vi "Error Handler.vi"(7 "function (unspecified)":T1, 8 "error in (no error)":errorcluster, 11 "errno":T2) -> (0 "error out":errorcluster)   [LabVIEW 2013, in "Linux RT IPC.lvlib" / "Pipes.lvlib"]
uses:
  Pipes.lvlib
  <vilib>/NI/NI Linux RT Errno/Controls/Public/errno.ctl
  Controls/functions.ctl
  <vilib>/NI/NI Linux RT Errno/Linux Errno.lvlib
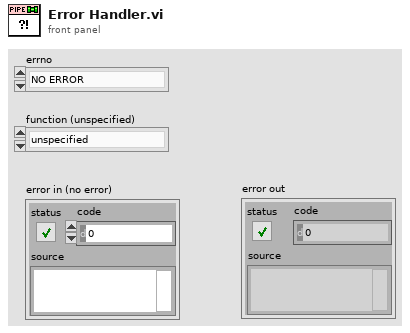
[diagram p1: front panel]
types:
  T1 = typedef "Linux RT IPC.lvlib/Pipes.lvlib/functions.ctl" = enum16{"unspecified", "mkfifo", "open", "read", "write", "close", "unlink"}
  T2 = typedef "Linux Errno.lvlib/errno.ctl" = enum16{"NO ERROR", "EPERM", "ENOENT", "ESRCH", "EINTR", "EIO", "ENXIO", "E2BIG", "ENOEXEC", "EBADF", "ECHILD", "EAGAIN", "ENOMEM", "EACCES", "EFAULT", "ENOTBLK", "EBUSY", "EEXIST", "EXDEV", "ENODEV", "ENOTDIR", "EISDIR", "EINVAL", "ENFILE", "EMFILE", "ENOTTY", "ETXTBSY", "EFBIG", "ENOSPC", "ESPIPE", "EROFS", "EMLINK", "EPIPE", "EDOM", "ERANGE", "EDADLK", "ENAMETOOLONG", "ENOLCK", "ENOSYS", "ENOTEMPTY", "ELOOP", "EWOULDBLOCK", "ENOMSG", "EIDRM", "ECHRNG", "EL2NSYNC", "EL3HLT", "EL3RST", "ELNRNG", "EUNATCH", "ENOCSI", "EL2HLT", "EBADE", "EBADR", "EXFULL", "ENOANO", "EBADRQC", "EBADSLT", "EDEADLOCK", "EBFONT", "ENOSTR", "ENODATA", "ETIME", "ENOSR", "ENONET", "ENOPKG", "EREMOTE", "ENOLINK", "EADV", "ESRMNT", "ECOMM", "EPROTO", "EMULTIHOP", "EDOTDOT", "EBADMSG", "EOVERFLOW", "ENOTUNIQ", "EBADFD", "EREMCHG", "ELIBACC", "ELIBBAD", "ELIBSCN", "ELIBMAX", "ELIBEXEC", "ELISEQ", "ERESTART", "ESTRPIPE", "EUSERS", "ENOTSOCK", "EDESTADDRREQ", "EMSGSIZE", "EPROTOTYPE", "ENOPROTOOPT", "EPROTONOSUPPORT", "ESOCKTNOSUPPORT", "EOPNOTSUPP", "EPFNOSUPPORT", "EAFNOSUPPORT", "EADDRINUSE", "EADDRNOTAVAIL", "ENETDOWN", "ENETUNREACH", "ENETRESET", "ECONNABORTED", "ECONNRESET", "ENOBUFS", "EISCONN", "ENOTCONN", "ESHUTDOWN", "ETOOMANYREFS", "ETIMEDOUT", "ECONNREFUSED", "EHOSTDOWN", "EHOSTUNREACH", "EALREADY", "EINPROGRESS", "ESTALE", "EUCLEAN", "ENOTNAM", "ENAVAIL", "EISNAM", "EREMOTEIO", "EDQUOT", "ENOMEDIUM", "EMEDIUMTYPE", "ECANCELED", "ENOKEY", "EKEYEXPIRED", "EKEYREVOKED", "EKEYREJECTED", "EOWNERDEAD", "ENOTRECOVERABLE", "ERFKILL", "EHWPOISON", "UNDEFINED"}
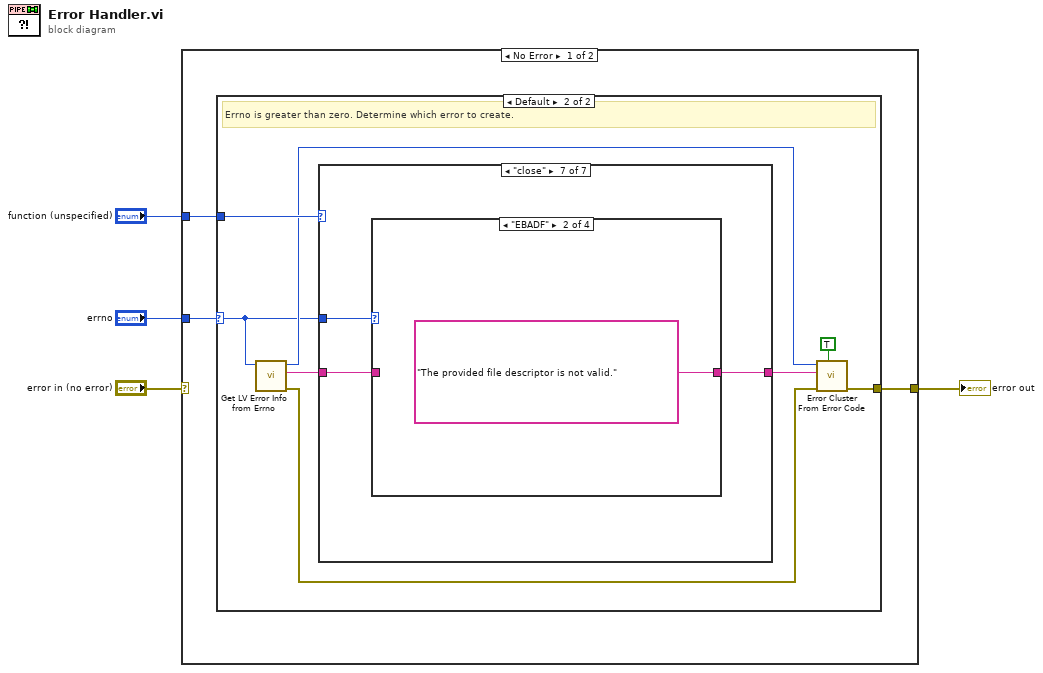
[diagram p0: block diagram]
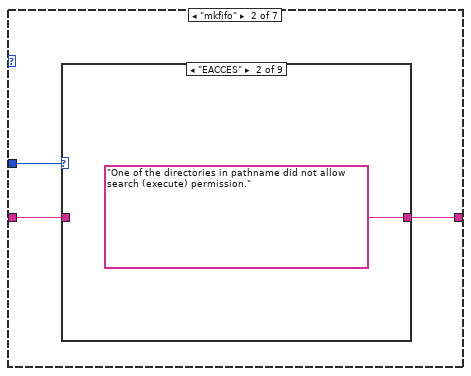
[diagram p4: hidden frame]
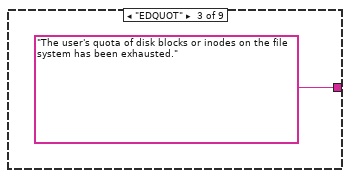
[diagram p6: hidden frame]
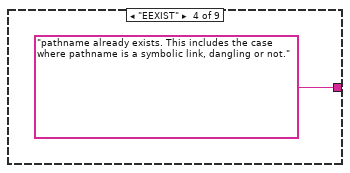
[diagram p7: hidden frame]
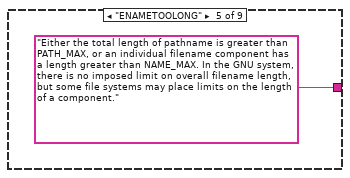
[diagram p8: hidden frame]
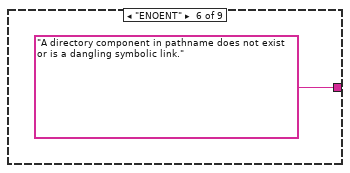
[diagram p9: hidden frame]
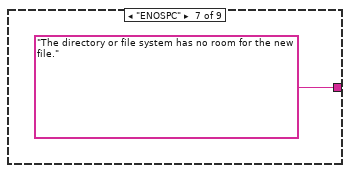
[diagram p10: hidden frame]
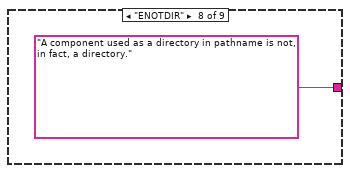
[diagram p11: hidden frame]
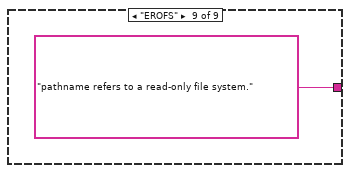
[diagram p12: hidden frame]
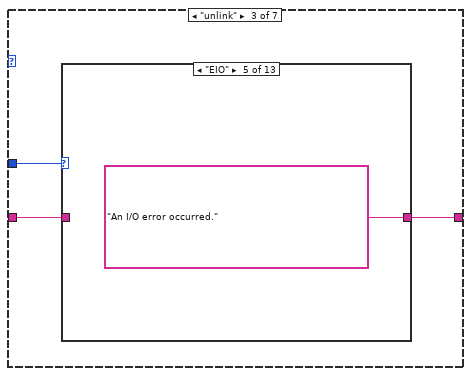
[diagram p13: hidden frame]
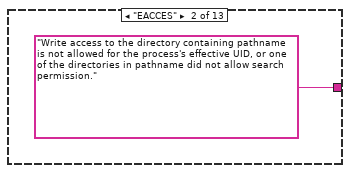
[diagram p15: hidden frame]
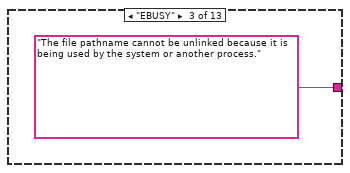
[diagram p16: hidden frame]
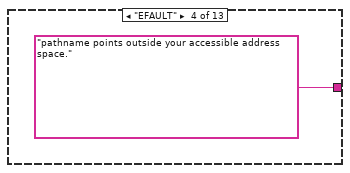
[diagram p17: hidden frame]
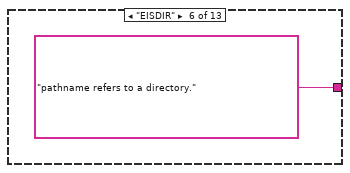
[diagram p18: hidden frame]
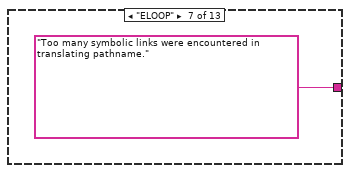
[diagram p19: hidden frame]
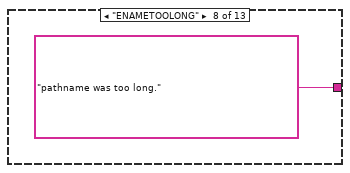
[diagram p20: hidden frame]
diagram:
  n1 = case shown="No Error" "error in (no error)" {
    selector: "error in (no error)" -> [_ w106]
    tunnel: [w7 w106] -> w3
    tunnel: "errno" -> [w5 _]
    tunnel: "function (unspecified)" -> [w6 _]
    frame No Error {
      n2 = case shown="Default" w5 {
        selector: w5 -> [_ w8]
        tunnel: [_ w15] -> w7
        tunnel: w6 -> [_ w13]
        frame "NO ERROR" {
          # "Errno is zero. No error occurred."
        }
        frame Default {
          # "Errno is greater than zero. Determine which error to create."
          n3 = call <vilib>:"Get LV Error Info from Errno.vi"("errno"=w8) -> ("error out"=w9:errorcluster, "error description"=w10:string, "error code"=w11:i32)  [unwired: 8 in]
          n4 = case shown="\"close\"" w13 {
            tunnel: w8 -> [_ w19 w31 w47 w74 w86 w101]
            tunnel: [w16 w18 w30 w46 w73 w85 w100] -> w12
            tunnel: w10 -> [w16 w17 w29 w45 w72 w84 w99]
            frame "unspecified", Default {
              # "No specific function was specified, so use generic error description."
            }
            frame "mkfifo" {
              n5 = case shown="\"EACCES\"" w19 {
                tunnel: [w20 "One of the directories in pathname did not allow search (execute) permission." "The user's quota of disk blocks or inodes on the file system has been exhausted." "pathname already exists. This includes the case where pathname is a symbolic link, dangling or not." "Either the total length of pathname is greater than PATH_MAX, or an individual filename component has a length greater than NAME_MAX. In the GNU system, there is no imposed limit on overall filename length, but some file systems may place limits on the length of a component." "A directory component in pathname does not exist or is a dangling symbolic link." "The directory or file system has no room for the new file." "A component used as a directory in pathname is not, in fact, a directory." "pathname refers to a read-only file system."] -> w18
                tunnel: w17 -> [w20 _ _ _ _ _ _ _ _]
                frame "NO ERROR", Default {
                }
                frame "EACCES" {
                }
                frame "EDQUOT" {
                }
                frame "EEXIST" {
                }
                frame "ENAMETOOLONG" {
                }
                frame "ENOENT" {
                }
                frame "ENOSPC" {
                }
                frame "ENOTDIR" {
                }
                frame "EROFS" {
                }
              }
            }
            frame "unlink" {
              n6 = case shown="\"EIO\"" w31 {
                tunnel: [w32 "Write access to the directory containing pathname is not allowed for the process's effective UID, or one of the directories in pathname did not allow search permission." "The file pathname cannot be unlinked because it is being used by the system or another process." "pathname points outside your accessible address space." "An I/O error occurred." "pathname refers to a directory." "Too many symbolic links were encountered in translating pathname." "pathname was too long." "A component in pathname does not exist or is a dangling symbolic link, or pathname is empty." "Insufficient kernel memory was available." "A component used as a directory in pathname is not, in fact, a directory." "The system does not allow unlinking of directories, or unlinking of directories requires privileges that the calling process doesn't have. Or, the file system does not allow unlinking of files." "pathname refers to a file on a read-only file system."] -> w30
                tunnel: w29 -> [w32 _ _ _ _ _ _ _ _ _ _ _ _]
                frame "NO ERROR", Default {
                }
                frame "EACCES" {
                }
                frame "EBUSY" {
                }
                frame "EFAULT" {
                }
                frame "EIO" {
                }
                frame "EISDIR" {
                }
                frame "ELOOP" {
                }
                frame "ENAMETOOLONG" {
                }
                frame "ENOENT" {
                }
                frame "ENOMEM" {
                }
                frame "ENOTDIR" {
                }
                frame "EPERM" {
                }
                frame "EROFS" {
                }
              }
            }
            frame "open" {
              n7 = case shown="\"EWOULDBLOCK\"" w47 {
                tunnel: [w48 "The requested access to the file is not allowed, or search permission is denied for one of the directories in the path prefix of pathname, or the file did not exist yet and write access to the parent directory is not allowed." "Where O_CREAT is specified, the file does not exist, and the user's quota of disk blocks or inodes on the file system has been exhausted." "pathname already exists and O_CREAT and O_EXCL were used." "pathname points outside your accessible address space." "pathname refers to a regular file that is too large to be opened. The usual scenario here is that an application compiled on a 32-bit platform without -D_FILE_OFFSET_BITS=64 tried to open a file whose size exceeds (2<<31)-1 bits." "While blocked waiting to complete, the call was interrupted by a signal handler." "The file descriptor does not reference a regular file." "pathname refers to a directory and the access requested involved writing (that is, O_WRONLY or O_RDWR is set)." "Too many symbolic links were encountered in resolving pathname." "The process already has the maximum number of files open." "pathname was too long." "The system limit on the total number of open files has been reached." "pathname refers to a device special file and no corresponding device exists." "The named file does not exist." "Insufficient kernel memory was available." "pathname was to be created but the device containing pathname has no room for the new file." "A component used as a directory in pathname is not, in fact, a directory." "O_NONBLOCK | O_WRONLY is set, the named file is a FIFO and no process has the file open for reading. Or, the file is a device special file and no corresponding device exists." "pathname refers to a regular file that is too large to be opened. The usual scenario here is that an application compiled on a 32-bit platform without -D_FILE_OFFSET_BITS=64 tried to open a file whose size exceeds (2<<31)-1 bits." "The O_NOATIME flag was specified, but the effective user ID of the caller did not match the owner of the file and the caller was not privileged (CAP_FOWNER)." "pathname refers to a file on a read-only file system and write access was requested." "pathname refers to an executable image which is currently being executed and write access was requested." "The O_NONBLOCK flag was specified, and an incompatible lease was held on the file."] -> w46
                tunnel: w45 -> [w48 _ _ _ _ _ _ _ _ _ _ _ _ _ _ _ _ _ _ _ _ _ _ _]
                frame "NO ERROR", Default {
                }
                frame "EACCES" {
                }
                frame "EDQUOT" {
                }
                frame "EEXIST" {
                }
                frame "EFAULT" {
                }
                frame "EFBIG" {
                }
                frame "EINTR" {
                }
                frame "EINVAL" {
                }
                frame "EISDIR" {
                }
                frame "ELOOP" {
                }
                frame "EMFILE" {
                }
                frame "ENAMETOOLONG" {
                }
                frame "ENFILE" {
                }
                frame "ENODEV" {
                }
                frame "ENOENT" {
                }
                frame "ENOMEM" {
                }
                frame "ENOSPC" {
                }
                frame "ENOTDIR" {
                }
                frame "ENXIO" {
                }
                frame "EOVERFLOW" {
                }
                frame "EPERM" {
                }
                frame "EROFS" {
                }
                frame "ETXTBSY" {
                }
                frame "EWOULDBLOCK" {
                }
              }
            }
            frame "read" {
              n8 = case shown="\"EINVAL\"" w74 {
                tunnel: [w75 "The file descriptor fd refers to a file other than a socket and has been marked nonblocking (O_NONBLOCK), and the read would block." "The file descriptor fd refers to a file other than a socket and has been marked nonblocking (O_NONBLOCK), and the read would block." "fd is not a valid file descriptor or is not open for reading." "buf is outside your accessible address space." "The call was interrupted by a signal before any data was read" "fd is attached to an object which is unsuitable for reading; or the file was opened with the O_DIRECT flag, and either the address specified in buf, the value specified in count, or the current file offset is not suitably aligned." "An I/O error occurred." "fd refers to a directory."] -> w73
                tunnel: w72 -> [w75 _ _ _ _ _ _ _ _]
                frame "NO ERROR", Default {
                }
                frame "EAGAIN" {
                }
                frame "EWOULDBLOCK" {
                }
                frame "EBADF" {
                }
                frame "EFAULT" {
                }
                frame "EINTR" {
                }
                frame "EINVAL" {
                }
                frame "EIO" {
                }
                frame "EISDIR" {
                }
              }
            }
            frame "write" {
              n9 = case shown="\"EPIPE\"" w86 {
                tunnel: [w87 "The file descriptor fd refers to a file other than a socket and has been marked nonblocking (O_NONBLOCK), and the write would block." "The file descriptor fd refers to a file other than a socket and has been marked nonblocking (O_NONBLOCK), and the write would block." "fd is not a valid file descriptor or is not open for writing." "fd refers to a datagram socket for which a peer address has not been set using connect(2)." "The user's quota of disk blocks on the file system containing the file referred to by fd has been exhausted." "buf is outside your accessible address space." "An attempt was made to write a file that exceeds the implementation-defined maximum file size or the process's file size limit, or to write at a position past the maximum allowed offset." "The call was interrupted by a signal before any data was written." "A low-level I/O error occurred while modifying the inode." "The device containing the file referred to by fd has no room for the data." "fd is connected to a pipe or socket whose reading end is closed. When this happens the writing process will also receive a SIGPIPE signal. (Thus, the write return value is seen only if the program catches, blocks or ignores this signal.)"] -> w85
                tunnel: w84 -> [w87 _ _ _ _ _ _ _ _ _ _ _]
                frame "NO ERROR", Default {
                }
                frame "EAGAIN" {
                }
                frame "EWOULDBLOCK" {
                }
                frame "EBADF" {
                }
                frame "EDESTADDRREQ" {
                }
                frame "EDQUOT" {
                }
                frame "EFAULT" {
                }
                frame "EFBIG" {
                }
                frame "EINTR" {
                }
                frame "EIO" {
                }
                frame "ENOSPC" {
                }
                frame "EPIPE" {
                }
              }
            }
            frame "close" {
              n10 = case shown="\"EBADF\"" w101 {
                tunnel: [w102 "The provided file descriptor is not valid." "The close() call was interrupted by a signal." "An I/O error occurred."] -> w100
                tunnel: w99 -> [w102 _ _ _]
                frame "NO ERROR", Default {
                }
                frame "EBADF" {
                }
                frame "EINTR" {
                }
                frame "EIO" {
                }
              }
            }
          }
          n11 = call <vilib>:"Error Cluster From Error Code.vi"("show call chain? (False)"=TRUE, "error in (no error)"=w9, "error message (\"\")"=w12, "error code (0)"=w11) -> ("error out"=w15:errorcluster)  [unwired: 5 in]
        }
      }
    }
    frame Error {
      # "Error already exists. Pass through."
    }
  }
  "error out" <- w3
